vi "Julian_project1.vi"() -> ()   [LabVIEW 2020]
uses:
  <vilib>/express/express arith-compare/Formula/XNode/ExpressFormulaBlockNode.xnode
panel:
  in  "Degrees - Radians":bool
  in  "Y":dbl
  in  "X":dbl
  in  "stop":bool
  in  "Function":T1(ring)
  out "Answer":dbl
  in  "Input 2":dbl
  in  "Input 1":dbl
  # "="
  # "The following panel is a simple calculator that \nadds, subtracts, multiplies, divides and performs the \nfollowing functions: Power, square root, cos, sin, and \ntan.\n\nThe inputs are labeled input 1 and 2. You can select your \nfunction using the function box.  \n\nFor cos, sin, and tan functions, you can select degrees or radians.\nThe input changes to degree or radians depending on the switch.\n\nThe stop function can be used to stop the program."
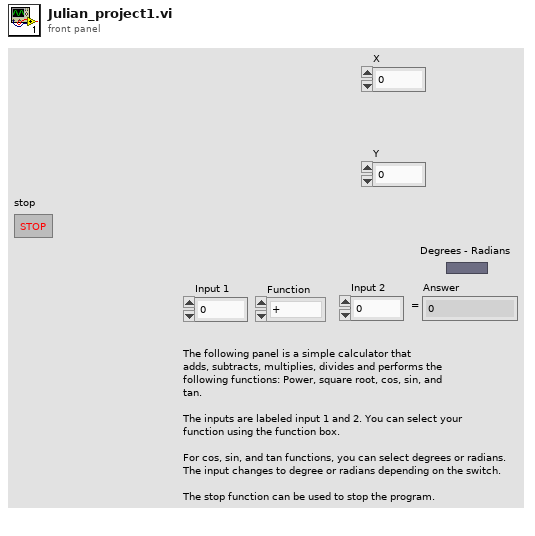
[diagram p1: front panel]
types:
  T1 = enum16{"+", "-", "/", "*", "^", "^ 1/2", "cos", "sin", "tan"}
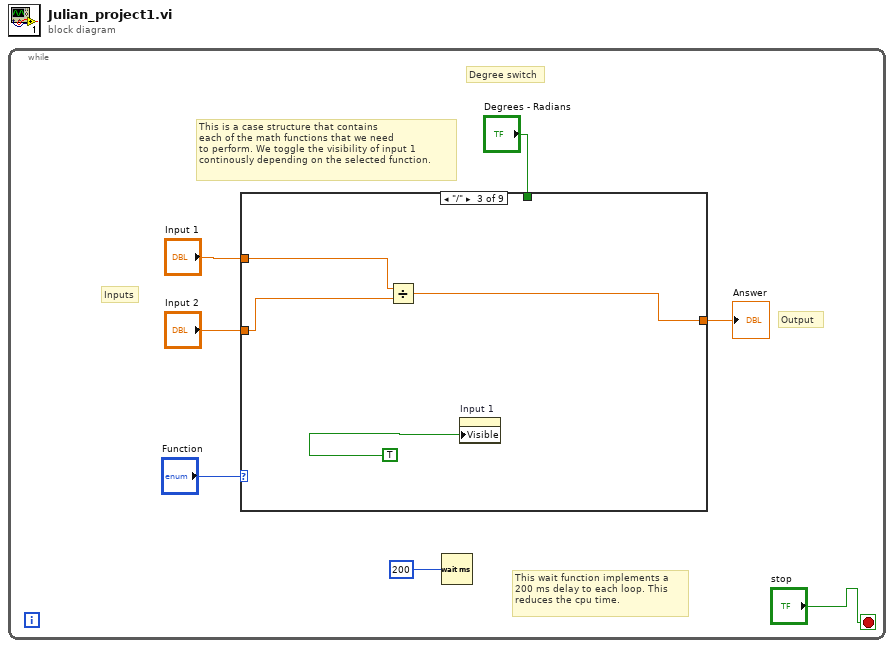
[diagram p0: block diagram]
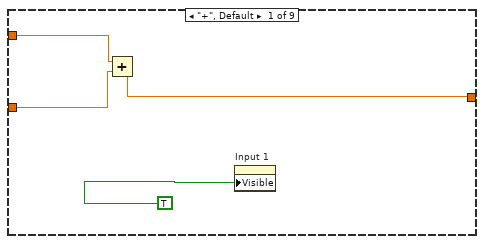
[diagram p2: hidden frame]
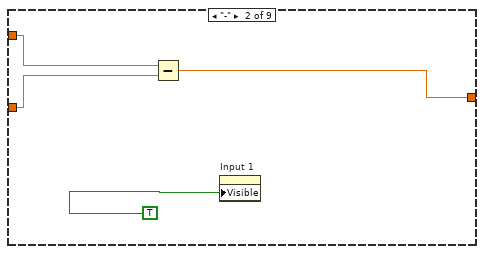
[diagram p3: hidden frame]
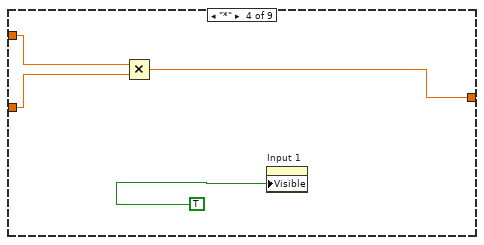
[diagram p4: hidden frame]
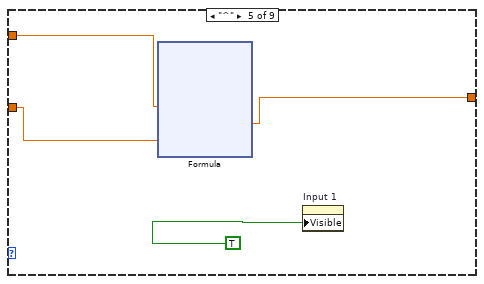
[diagram p5: hidden frame]
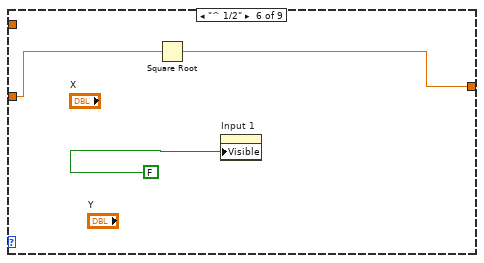
[diagram p6: hidden frame]
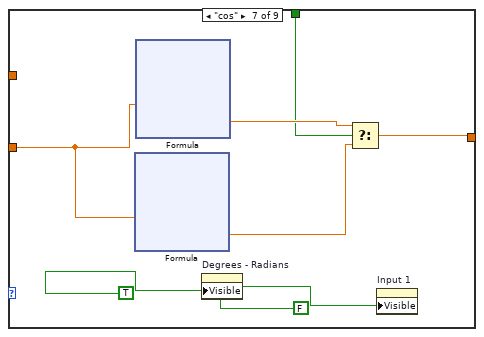
[diagram p7: hidden frame]
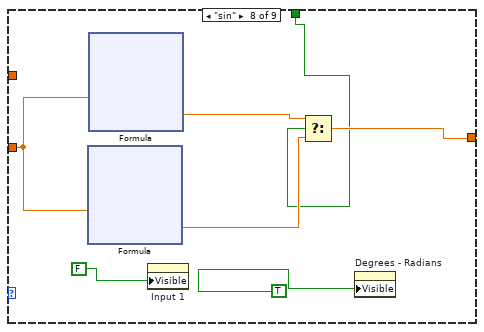
[diagram p8: hidden frame]
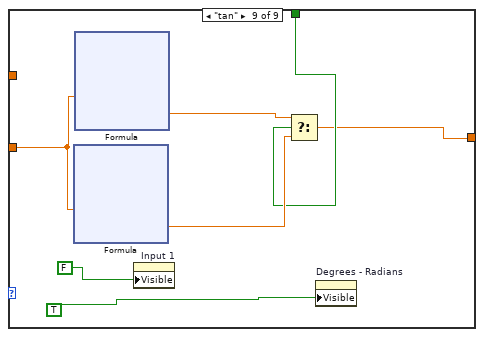
[diagram p9: hidden frame]
diagram:
  n1 = while {
    stop <- "stop" stop-if-true
    # "This is a case structure that contains\neach of the math functions that we need \nto perform. We toggle the visibility of input 1\ncontinously depending on the selected function."
    # "Output"
    # "This wait function implements a \n200 ms delay to each loop. This \nreduces the cpu time."
    # "Degree switch"
    # "Inputs"
    n2 = case shown="\"/\"" "Function" {
      tunnel: "Input 1" -> [w11 w15 w19 w23 w27 _ _ _ _]
      tunnel: "Input 2" -> [w10 w14 w18 w22 w26 w39 w43 w67 w87]
      tunnel: [w9 w13 w17 w21 w25 w40 w45 w66 w88] -> w4
      tunnel: "Degrees - Radians" -> [_ _ _ _ _ _ w42 w65 w89]
      frame "+", Default {
        n3 = Add(x=w11, y=w10) -> (x+y=w9:dbl)
        n4 = property on="Input 1" class="DigNum (strict)"("Visible"=TRUE) -> ()  [unwired: 2 in, 2 out]
      }
      frame "-" {
        n5 = Subtract(x=w15, y=w14) -> (x-y=w13:dbl)
        n6 = property on="Input 1" class="DigNum (strict)"("Visible"=TRUE) -> ()  [unwired: 2 in, 2 out]
      }
      frame "/" {
        n7 = Divide(x=w19, y=w18) -> (x/y=w17:dbl)
        n8 = property on="Input 1" class="DigNum (strict)"("Visible"=TRUE) -> ()  [unwired: 2 in, 2 out]
      }
      frame "*" {
        n9 = Multiply(x=w23, y=w22) -> (x*y=w21:dbl)
        n10 = property on="Input 1" class="DigNum (strict)"("Visible"=TRUE) -> ()  [unwired: 2 in, 2 out]
      }
      frame "^" {
        n11 = xnode "Formula"("X1"=w27, "X2"=w26) -> ("Result"=w25:dbl)  [unwired: 1 in, 1 out]
        n12 = property on="Input 1" class="DigNum (strict)"("Visible"=TRUE) -> ()  [unwired: 2 in, 2 out]
      }
      frame "^ 1/2" {
        n13 = Square Root(x=w39) -> (sqrt(x)=w40:dbl)
        n14 = property on="Input 1" class="DigNum (strict)"("Visible"=FALSE) -> ()  [unwired: 2 in, 2 out]
      }
      frame "cos" {
        n15 = xnode "Formula"("X1"=w43) -> ("Result"=w44:dbl)  [unwired: 1 in, 1 out]
        n16 = xnode "Formula"("X1"=w43) -> ("Result"=w46:dbl)  [unwired: 1 in, 1 out]
        n17 = property on="Degrees - Radians" class="Bool (strict)"("Visible"=TRUE) -> ()  [unwired: 2 in, 2 out]
        n18 = Select(t=w46, s=w42, f=w44) -> (s? t:f=w45:dbl)
        n19 = property on="Input 1" class="DigNum (strict)"("Visible"=FALSE) -> ()  [unwired: 2 in, 2 out]
      }
      frame "sin" {
        n20 = xnode "Formula"("X1"=w67) -> ("Result"=w69:dbl)  [unwired: 1 in, 1 out]
        n21 = xnode "Formula"("X1"=w67) -> ("Result"=w70:dbl)  [unwired: 1 in, 1 out]
        n22 = property on="Input 1" class="DigNum (strict)"("Visible"=FALSE) -> ()  [unwired: 2 in, 2 out]
        n23 = Select(t=w70, s=w65, f=w69) -> (s? t:f=w66:dbl)
        n24 = property on="Degrees - Radians" class="Bool (strict)"("Visible"=TRUE) -> ()  [unwired: 2 in, 2 out]
      }
      frame "tan" {
        n25 = xnode "Formula"("X1"=w87) -> ("Result"=w91:dbl)  [unwired: 1 in, 1 out]
        n26 = xnode "Formula"("X1"=w87) -> ("Result"=w92:dbl)  [unwired: 1 in, 1 out]
        n27 = property on="Input 1" class="DigNum (strict)"("Visible"=FALSE) -> ()  [unwired: 2 in, 2 out]
        n28 = Select(t=w92, s=w89, f=w91) -> (s? t:f=w88:dbl)
        n29 = property on="Degrees - Radians" class="Bool (strict)"("Visible"=TRUE) -> ()  [unwired: 2 in, 2 out]
      }
    }
    "Answer" <- w4
    n30 = Wait (ms)(milliseconds to wait=200) -> ()  [unwired: 1 out]
  }
